vi "Close.vi"(8 "error in (no error)":errorcluster caption="entrée d'erreur (pas d'erreur)", 11 "Class Multimeter Rigol DM3058 en entrée":refnum<class "Class Multimeter Rigol DM3058.lvclass">) -> (0 "error out":errorcluster caption="sortie d'erreur", 3 "Class Multimeter Rigol DM3058 en sortie":refnum<class "Class Multimeter Rigol DM3058.lvclass">)   [LabVIEW 2020, in "Library Instrument & Equipement.lvlib" / "Library Multimeter.lvlib" / "Class Multimeter Rigol DM3058.lvclass"]
uses:
  Class Multimeter Rigol DM3058.lvclass
  C:/Users/ngarcin/OneDrive - Altyor/Standard TB/Class/Multimeter/Multimeter (Default)/Class Multimeter (Default).lvclass
  Class Multimeter Rigol DM3058.lvclass/Class Multimeter Rigol DM3058.ctl
  RIGOL DM3058/RIGOL DM3058.lvlib
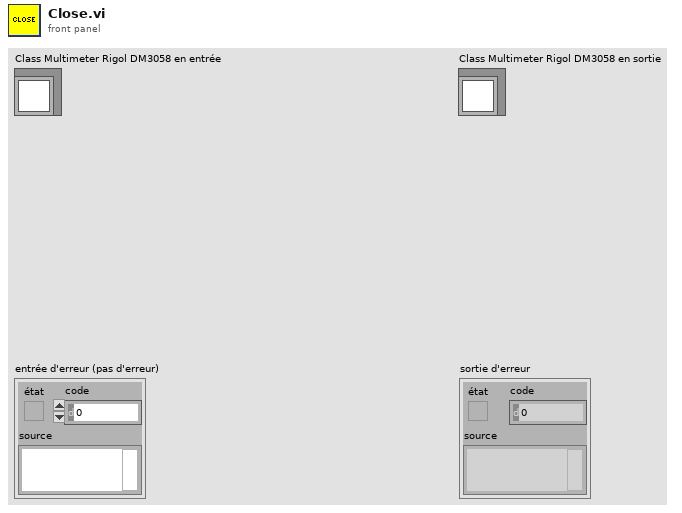
[diagram p1: front panel]
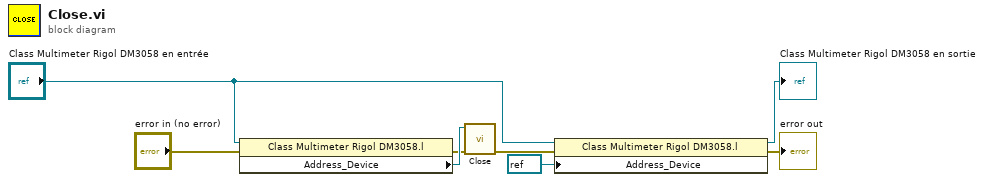
[diagram p0: block diagram]
diagram:
  n1 = property class="Class Multimeter Rigol DM3058.l"(reference="Class Multimeter Rigol DM3058 en entrée", error in="error in (no error)") -> (error out=w6:errorcluster, "Address_Device"=w7:refnum<visa-resource-name>)  [unwired: 1 out]
  n2 = call "Close.vi"("error in (no error)"=w6, "VISA resource name"=w7) -> ("error out"=w5:errorcluster)  [unwired: 9 in]
  n3 = property class="Class Multimeter Rigol DM3058.l"(reference="Class Multimeter Rigol DM3058 en entrée", error in=w5, "Address_Device"=refnum<visa-resource-name> refnum) -> (reference out=→"Class Multimeter Rigol DM3058 en sortie":refnum<class "Class Multimeter Rigol DM3058.lvclass">, error out=→"error out":errorcluster)
